vi "Process.vi"(8 "error in":errorcluster, 11 "Plugin in":refnum<class "Stereo Microphone Input.lvclass">) -> (0 "error out":errorcluster, 3 "Plugin out":refnum<class "Stereo Microphone Input.lvclass">)   [LabVIEW 2026, in "Stereo Microphone Input.lvlib" / "Stereo Microphone Input.lvclass"]
uses:
  Stereo Microphone Input.lvclass
  C:/Program Files/National Instruments/LabVIEW 2026/vi.lib/FlexLogger/SDK/PluginSDK.lvlibp/PEFClasses/SDK/Plugin/Plugin.lvclass
  Stereo Microphone Input.lvclass/Stereo Microphone Input.ctl
  <vilib>/FlexLogger/SDK/PluginSDK.lvlibp/PEFClasses/SDK/Plugin/DataHelpers/Write 2D DBL (NChan NSamples).vi
  C:/Program Files/National Instruments/LabVIEW 2026/vi.lib/FlexLogger/SDK/PluginSDK.lvlibp/PEFClasses/SDK/Processing Element/Processing Element.lvclass
  C:/Users/nkirchne/Documents/LabVIEW Projects/FlexLogger IO Plug-ins/Stereo Microphone Input/Stereo Microphone Input.lvclass
  <vilib>/FlexLogger/SDK/PluginSDK.lvlibp/PEFClasses/SDK/Plugin/Plugin.lvclass
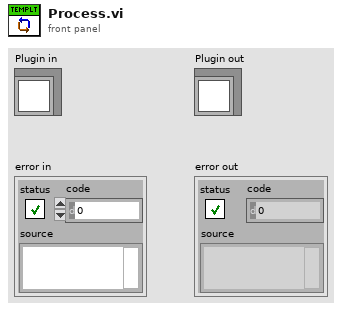
[diagram p1: front panel]
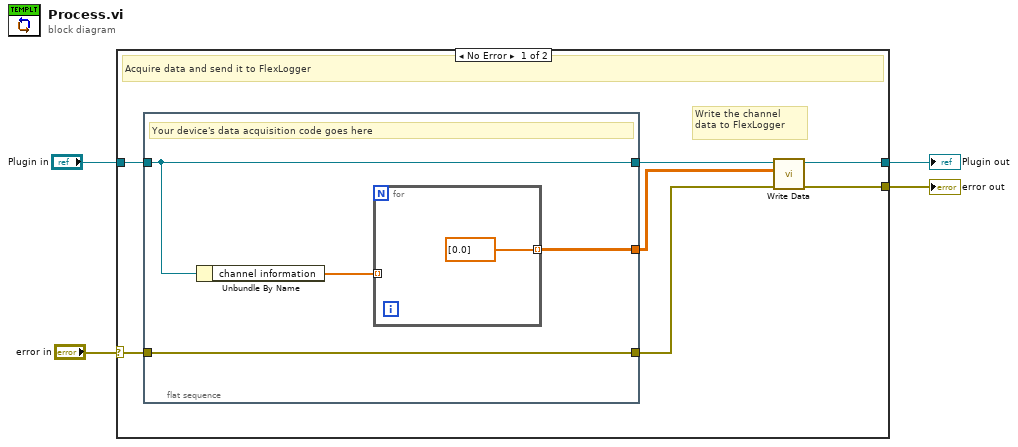
[diagram p0: block diagram]
diagram:
  n1 = case shown="No Error" "error in" {
    selector: "error in" -> [w10 w17]
    tunnel: [w6 w18] -> w4
    tunnel: "Plugin in" -> [w11 w18]
    tunnel: [w7 w17] -> w1
    frame No Error {
      # "Write the channel data to FlexLogger"
      # "Acquire data and send it to FlexLogger"
      n2 = flat-sequence {
        tunnel: [w14] -> w5
        tunnel: w11 -> [w13]
        tunnel: [w13] -> w9
        tunnel: w10 -> [w15]
        tunnel: [w15] -> w8
        frame #0 {
          # "Your device's data acquisition code goes here"
          n3 = Unbundle By Name(w13) -> ("channel information"=w12:dbl[])
          n4 = for {
            tunnel: [dbl[] [0.0]] -> w14 mode=indexing
            tunnel: w12 -> [_] mode=indexing
          }
        }
      }
      n5 = call-poly <vilib>:"Write Data.vi"("error in (no error)"=w8, "Data"=w5, "Plugin in"=w9) -> ("error out"=w7:errorcluster, "Plugin out"=w6:refnum<class "Stereo Microphone Input.lvclass">)  [unwired: 7 in]
    }
    frame Error {
    }
  }
  "error out" <- w1
  "Plugin out" <- w4
